vi "ItemSelection_ObtainSelectionQueue.vi"(8 "error in (no error)":errorcluster) -> (0 "error out":errorcluster, 2 "queue out":refnum<queue>)   [LabVIEW 2014, in "ItemSelection.lvlib"]
uses:
  ItemSelection.lvlib
  ItemSelection_Data.ctl
  ItemSelection_Command.ctl
  <resource>/Framework/Providers/API/ItemRef.ctl
  ItemSelection_NamesGlobal.vi
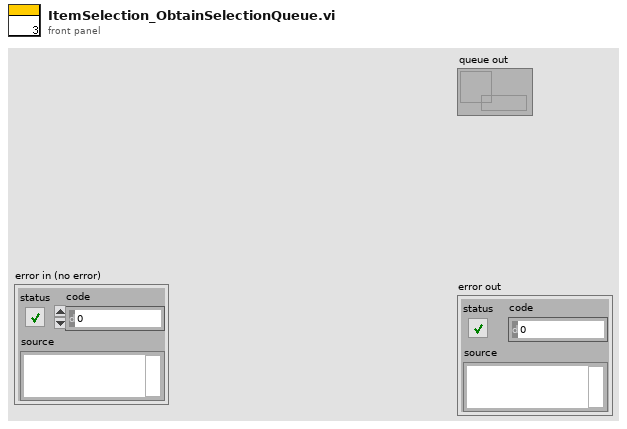
[diagram p1: front panel]
types:
  T1 = typedef "ItemSelection.lvlib/ItemSelection_Data.ctl" = cluster{"Command":T2, "Item Ref":T3}
  T2 = typedef "ItemSelection.lvlib/ItemSelection_Command.ctl" = enum16{"ItemSelected", "ItemUnselected"}
  T3 = typedef "ItemRef.ctl" = u64
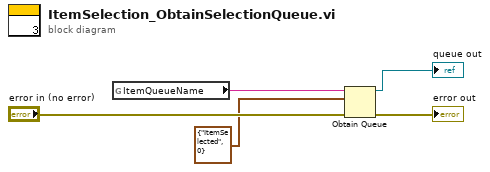
[diagram p0: block diagram]
diagram:
  n1 = global read "ItemSelection_NamesGlobal.vi" "ItemQueueName"() -> (w5:string)
  n2 = Obtain Queue(name (unnamed)=w5, element data type=T1 {"Command"=enum."ItemSelected", "Item Ref"=0} ("Data"), error in (no error)="error in (no error)") -> (queue out=→"queue out":refnum<queue>, error out=→"error out":errorcluster)  [unwired: 2 in, 1 out]
